vi "Action Reset Max-Min.vi"(0 "VISA resource name":refnum<visa-resource-name>, 7 "Reset Max/Min (T: Reset)":bool=TRUE, 11 "error in (no error)":errorcluster) -> (4 "VISA resource name out":refnum<visa-resource-name>, 15 "error out":errorcluster)   [LabVIEW 2019, in "Lake Shore Cryotronics 340.lvlib"]
doc: "This VI resets Min/Max function for all inputs."
uses:
  Lake Shore Cryotronics 340.lvlib
panel:
  # "Reset Max/Min\nDon't Reset Max/Min"
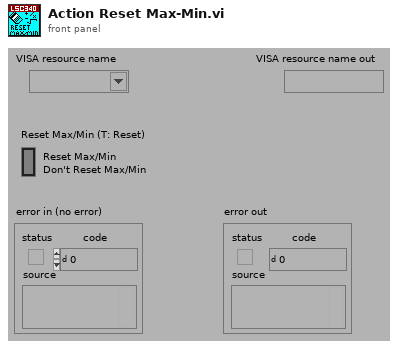
[diagram p1: front panel]
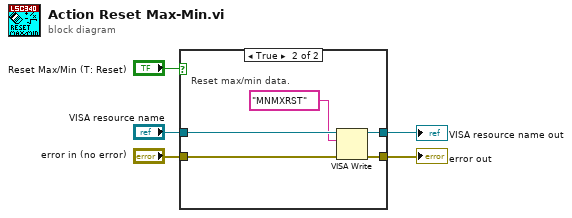
[diagram p0: block diagram]
diagram:
  n1 = case shown="True" "Reset Max/Min (T: Reset)" {
    tunnel: "VISA resource name" -> [w7 w12]
    tunnel: "error in (no error)" -> [w6 w11]
    tunnel: [w7 w10] -> w2
    tunnel: [w6 w9] -> w1
    frame False {
      # "Do not reset max/min."
    }
    frame True {
      # "Reset max/min data."
      n2 = VISA Write(VISA resource name=w12, write buffer="MNMXRST", error in (no error)=w11) -> (VISA resource name out=w10:refnum<visa-resource-name>, error out=w9:errorcluster)  [unwired: 1 out]
    }
  }
  "VISA resource name out" <- w2
  "error out" <- w1
